vi "例10.3  利用底层函数采集N幅图像 （设置参数）.vi"() -> ()   [LabVIEW 2012]
doc: "The Low-Level Sequence VI acquires a sequence of images and displays the images in an image control using low-level acquisition VIs. A sequence is appropriate for applications in which you want to process multiple images."
uses:
  <vilib>/userdefined/High Color/IMAQdx.ctl
  <vilib>/vision/driver/IMAQdx.llb/IMAQdx Acquisition Mode.ctl
  <vilib>/vision/driver/IMAQdx.llb/IMAQdx Buffer Number Mode.ctl
  <vilib>/vision/driver/NI_Vision_Acquisition_Software.lvlib
  <resource>/objmgr/imaqdx.rc
panel:
  in  "Camera Name":T1
  out "Image Array":T2[](array[plugin-control])
  in  "Number of Images":u32=5
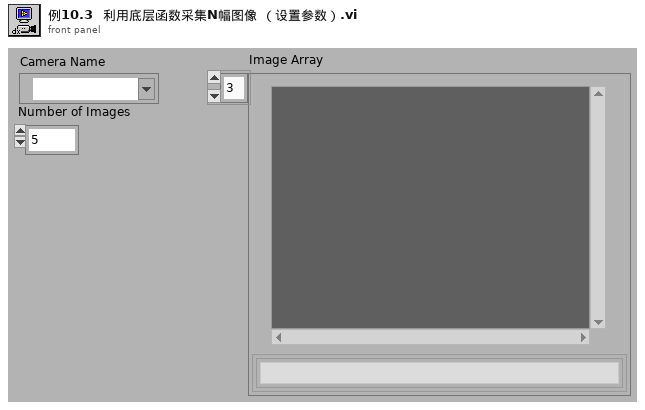
[diagram p1: front panel]
types:
  T1 = typedef "IMAQdx.ctl" = refnum<k21>
  T2 = typedef "IMAQ Image.ctl" = refnum<image>
  T3 = typedef "NI_Vision_Acquisition_Software.lvlib/IMAQdx Acquisition Mode.ctl" = enum32{"One Shot", "Continuous"}
  T4 = typedef "NI_Vision_Acquisition_Software.lvlib/IMAQdx Buffer Number Mode.ctl" = enum32{"Next", "Last", "Buffer Number"}
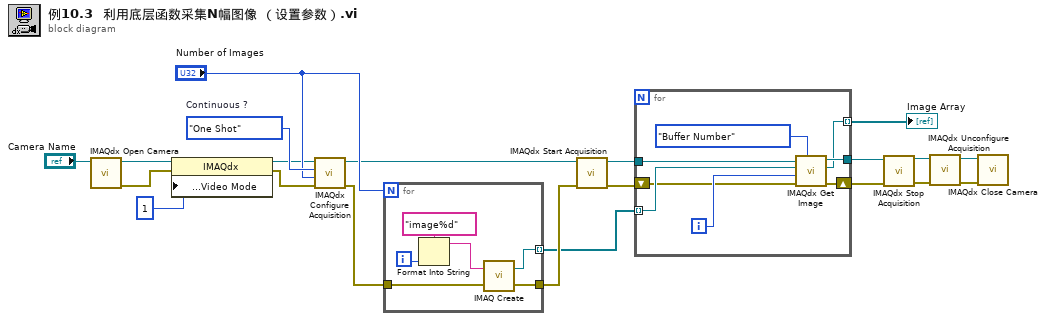
[diagram p0: block diagram]
diagram:
  w20 = IMAQdx_Acquisition_Mode."One Shot"  # Continuous ?
  n1 = call <vilib>:"IMAQdx Open Camera.vi"("Session In"="Camera Name") -> ("error out"=w4:errorcluster, "Session Out"=w5:T1)  [unwired: 2 in, 7 out]
  n2 = property class="IMAQdx"(reference=w5, error in=w4, "Acquisition Attributes:Video Mode"=u32 1 ("VideoMode")) -> (reference out=w3:T1, error out=w2:errorcluster)
  n3 = call <vilib>:"IMAQdx Configure Acquisition.vi"("error in"=w2, "Number of Buffers"="Number of Images", "Continuous?"=w20, "Session In"=w3) -> ("error out"=w18:errorcluster, "Session Out"=w17:T1)  [unwired: 6 out]
  n4 = for {
    N: "Number of Images" -> [_]
    tunnel: w18 -> [w27]
    tunnel: [w26] -> w14 mode=indexing
    tunnel: [w25] -> w16
    i -> [w24]
    n5 = Format Into String(format string="image%d" ("Image Name"), w24) -> (resulting string=w23:string)  [unwired: 2 in, 1 out]
    n6 = call "IMAQ Create"("Image Name"=w23, "error in (no error)"=w27) -> ("New Image"=w26:T2, "error out"=w25:errorcluster)  [unwired: 2 in, 1 out]
  }
  n7 = call <vilib>:"IMAQdx Start Acquisition.vi"("error in"=w16, "Session In"=w17) -> ("error out"=w13:errorcluster, "Session Out"=w15:T1)  [unwired: 8 out]
  n8 = for {
    tunnel: w14 -> [w34] mode=indexing
    shift-right: [w32] -> w12
    shift-left: w13 -> [w33]
    tunnel: [w31] -> w11
    tunnel: w15 -> [w30]
    tunnel: [w28] -> w6 mode=indexing
    i -> [w35]
    n9 = call <vilib>:"IMAQdx Get Image.vi"("Buffer Number Mode (Next)"=IMAQdx_Buffer_Number_Mode."Buffer Number", "error in"=w33, "Buffer Number In"=w35, "Image In"=w34, "Session In"=w30) -> ("error out"=w32:errorcluster, "Image Out"=w28:T2, "Session Out"=w31:T1)  [unwired: 4 out]
  }
  "Image Array" <- w6
  n10 = call <vilib>:"IMAQdx Stop Acquisition.vi"("error in"=w12, "Session In"=w11) -> ("error out"=w10:errorcluster, "Session Out"=w9:T1)  [unwired: 8 out]
  n11 = call <vilib>:"IMAQdx Unconfigure Acquisition.vi"("error in"=w10, "Session In"=w9) -> ("error out"=w8:errorcluster, "Session Out"=w7:T1)  [unwired: 8 out]
  n12 = call <vilib>:"IMAQdx Close Camera.vi"("error in"=w8, "Session In"=w7) -> ()  [unwired: 10 out]
